vi "Actor Core.vi"(8 "error in":errorcluster, 11 "DAQ DI in":refnum<class "DAQ DI.lvclass">) -> (0 "error out":errorcluster, 3 "Actor out":refnum<class "Actor.lvclass">)   [LabVIEW 2020, in "DAQ DI.lvlib" / "DAQ DI.lvclass"]
doc: "<p>(<strong>Filename</strong>: <span class=\"dnl\">Actor Framework.lvlib:Actor.lvclass:Actor Core.vi</span>)</p>\n<p>Receives messages to the actor, reacts to them, and initiates any error handling that may shut the actor down.</p>\n<p>Descendant classes may override this VI to append parallel tasks for the actor to complete while it handles messages. Overrides use the <a href=\"nihelplauncher://docs/csh?context=lvcore_glang_udclass\">Call Parent Class Method</a> node.</p>"
uses:
  DAQ DI.lvclass
  DAQ DI.lvclass/DAQ DI.ctl
  C:/Program Files (x86)/National Instruments/LabVIEW 2026/vi.lib/ActorFramework/Actor/Actor.lvclass
  C:/Users/taacr/OneDrive/HP/Local/Actor Framework/DAQ DI/DAQ DI/DAQ DI.lvclass
  <vilib>/ActorFramework/Actor/Actor.lvclass
  Supervisor/Supervisor Messages/Acquire Status Msg/Acquire Status Msg.lvclass
panel:
  out "Status":u8
  out "DAQmx Digital Channel":tag
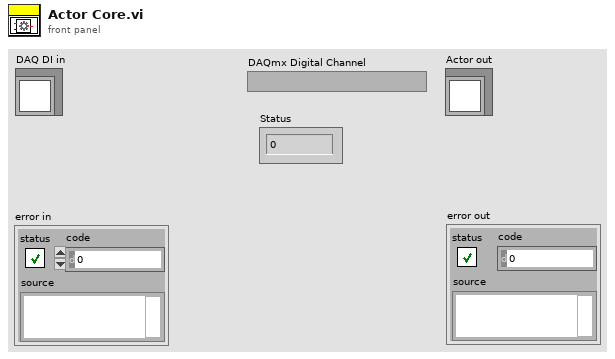
[diagram p1: front panel]
types:
  T1 = typedef "DAQ DI.lvlib/DAQ DI.lvclass/User Events.ctl" = cluster{"Stop Event":refnum<user-event>, "DAQmx Digital Channel Event":refnum<user-event>, "Status Event":refnum<user-event>}
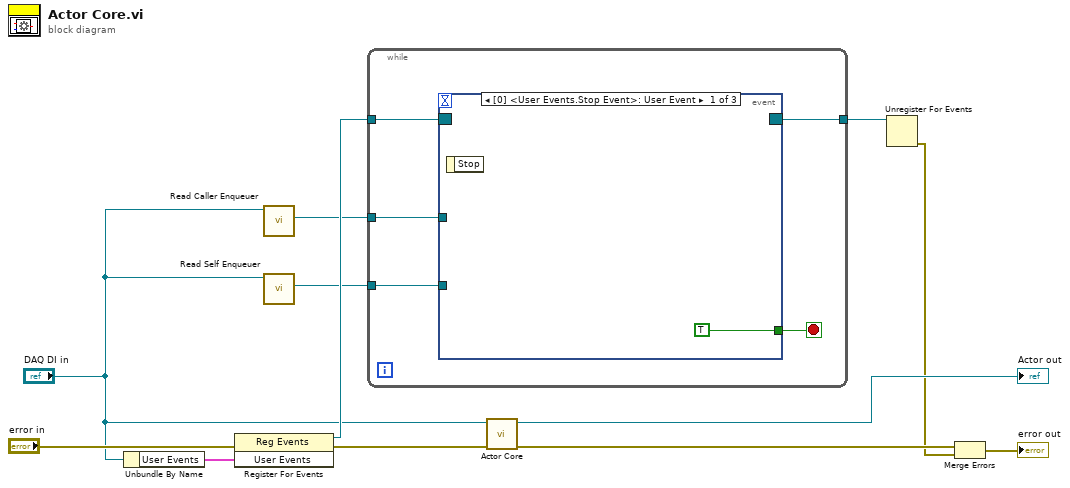
[diagram p0: block diagram]
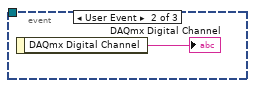
[diagram p2: hidden frame]
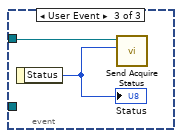
[diagram p3: hidden frame]
diagram:
  n1 = Unbundle By Name("DAQ DI in") -> ("User Events"=w11:T1)
  n2 = register-events(error in="error in", w11) -> (reference out=w8:refnum<event-registration>, error out=w9:errorcluster)  [unwired: 1 in]
  n3 = call <vilib>:"Read Caller Enqueuer.vi"("Actor"="DAQ DI in") -> ("Caller Enqueuer"=w6:refnum<class "Message Enqueuer.lvclass">)  [unwired: 10 in]
  n4 = call <vilib>:"Read Self Enqueuer.vi"("Actor"="DAQ DI in") -> ("Self Enqueuer"=w5:refnum<class "Message Enqueuer.lvclass">)  [unwired: 10 in]
  n5 = while {
    tunnel: w8 -> [w17]
    tunnel: w6 -> [w16]
    tunnel: w5 -> [w15]
    tunnel: [w14] -> w4
    stop <- w13 stop-if-true
    n6 = event shown="[0] <User Events.Stop Event>: User Event" {
      selector: w17 -> [_ _ _]
      dyn-events: [_ _ _] -> w14
      timeout: _ -> [_ _ _]
      tunnel: w16 -> [_ _ w21]
      tunnel: w15 -> [_ _ _]
      tunnel: [TRUE _ _] -> w13
      event User Event {
        n7 = event-data() -> ()  [unwired: 1 in, 1 out]
      }
      event User Event {
        n8 = event-data() -> ("DAQmx Digital Channel"=→"DAQmx Digital Channel":tag)  [unwired: 1 in]
      }
      event User Event {
        n9 = event-data() -> ("Status"=w20:u8)  [unwired: 1 in]
        "Status" <- w20
        n10 = call "Send Acquire Status.vi"("Status"=w20, "Message Enqueuer"=w21) -> ()  [unwired: 8 in, 2 out]
      }
    }
  }
  n11 = call-parent "Actor Core.vi"("error in"=w9, "Actor in"="DAQ DI in") -> ("error out"=w3:errorcluster, "Actor out"=→"Actor out":refnum<class "Actor.lvclass">)  [unwired: 8 in]
  n12 = Unregister For Events(event registration refnum=w4) -> (error out=w2:errorcluster)  [unwired: 1 in]
  n13 = Merge Errors(w3, w2) -> (→"error out":errorcluster)
